vi "XNET Bus Monitor Redux.vi"() -> ()   [LabVIEW 2025, in "XNET Bus Monitor Client.lvlib"]
uses:
  XNET Bus Monitor Client.lvlib
  xnet_can_bus_monitor_api_client/RPC Messages/ni_xnet_can_bm_api_FrameFilter.ctl
  xnet_can_bus_monitor_api_client/RPC Messages/ni_xnet_can_bm_api_DirectionFilter.ctl
  Types/GUI.StateVariables.ctl
  Types/GUI.Controls.Refs.ctl
  Types/StreamEngine.QueueRefs.ctl
  Types/StreamEngine.CmdQueueData.ctl
  Types/StreamEngine.CmdQueueData.Cmd.ctl
  Types/SubProcessEngine.QueueRefs.ctl
  Types/SubProcessEngine.CmdQueueData.ctl
  Types/SubProcessEngine.CmdQueueData.Cmd.ctl
  Types/gRPC.ConnectionInfo.ctl
  <vilib>/gRPC/LabVIEW gRPC Library/Shared/grpcId.ctl
  Types/StreamEngine.State.ctl
  Types/SubProcessEngine.State.ctl
  Types/StreamEngine.CmdQueueData.InitialSettings.ctl
  xnet_can_bus_monitor_api_client/RPC Messages/ni_xnet_can_bm_api_StreamBusReply.ctl
  xnet_can_bus_monitor_api_client/RPC Messages/ni_xnet_can_bm_api_CanCommState.ctl
  xnet_can_bus_monitor_api_client/RPC Messages/ni_xnet_can_bm_api_CommState.ctl
  xnet_can_bus_monitor_api_client/RPC Messages/ni_xnet_can_bm_api_LastCommError.ctl
  xnet_can_bus_monitor_api_client/RPC Messages/ni_xnet_can_bm_api_Frame.ctl
  xnet_can_bus_monitor_api_client/RPC Messages/ni_xnet_can_bm_api_ErrorInfo.ctl
  Types/SubProcessEngine.CmdQueueData.Publish.ctl
  Types/StreamEngine.Parameters.ctl
  xnet_can_bus_monitor_api_client/RPC Messages/ni_xnet_can_bm_api_FilterInfo.ctl
  xnet_can_bus_monitor_api_client/RPC Messages/ni_xnet_can_bm_api_PassThruRequest.ctl
  xnet_can_bus_monitor_api_client/RPC Messages/ni_xnet_can_bm_api_SetStreamingFilterRequest.ctl
  <vilib>/Utility/miscctls.llb/LVRowAndColumnUnsignedTypeDef.ctl
  <vilib>/dlg_ctls.llb/Space Constant.vi
  SubVIs/Convert.BusDataArrayToStringArray.vi
  <vilib>/Utility/error.llb/Trim Whitespace.vi
  SubVIs/Convert.TimeToUTCString.vi
  <vilib>/Utility/error.llb/Trim Whitespace One-Sided.vi
  <vilib>/Utility/libraryn.llb/Check if File or Folder Exists.vi
  <vilib>/Utility/libraryn.llb/Get File Extension.vi
  <userlib>/_OpenG.lib/array/array.llb/Sort Array__ogtk.vi
  <userlib>/_OpenG.lib/array/array.llb/Sort 2D Array (String)__ogtk.vi
  xnet_can_bus_monitor_api_client/RPC Service/NI_XNET_CAN_Bus_Monitor_API/Begin NI_XNET_CAN_Bus_Monitor_API StreamBus.vi
  xnet_can_bus_monitor_api_client/RPC Service/NI_XNET_CAN_Bus_Monitor_API/End NI_XNET_CAN_Bus_Monitor_API StreamBus.vi
  xnet_can_bus_monitor_api_client/xnet_can_bus_monitor_api_client.lvlib
  <vilib>/gRPC/LabVIEW gRPC Library/grpc-lvsupport-release.lvlib
panel:
  out "error out":errorcluster
  out "Device":string
  in  "Tab Control":enum32{"Bus Stream", "RAW"}(tab)
  out "Log Status":string
  in  "Direction Filter":T1
  in  "Type Filter":T2
  in  "Reset Filter":bool
  in  "Host Filter":bool
  in  "Filter IDs":string caption="Filter IDs (format = x<ID>, comma separated, ID x0 = Bus Error)"
  in  "Clear History":bool
  out "Table Control":string[][](table)
  in  "Sort By ID":bool
  out "Stream Connected":bool
  out "Bus Status":string
  in  "Log":bool
  in  "Pause":bool
  in  "Extended?":bool
  in  "Identifier":u32 format="%x"
  in  "Raw Bytes":u8[](array[numeric])
  in  "Type":T3(ring)
  out "Error":errorcluster
  in  "Clear Raw":bool
  in  "Send Raw":bool
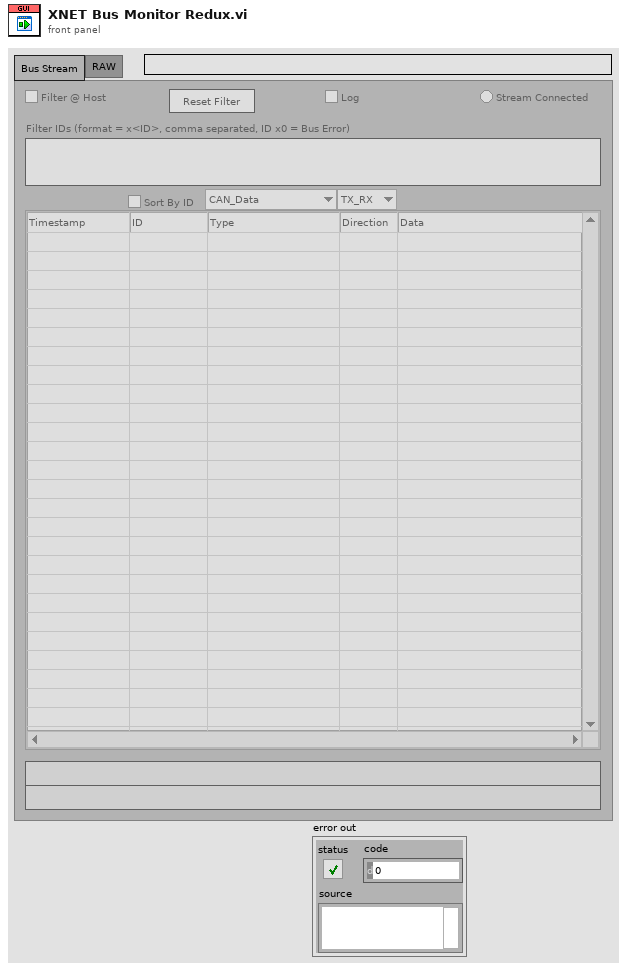
[diagram p1: front panel]
types:
  T1 = typedef "xnet_can_bus_monitor_api_client.lvlib/ni_xnet_can_bm_api_DirectionFilter.ctl" = enum32{"TX_RX", "RX", "TX"}
  T2 = typedef "xnet_can_bus_monitor_api_client.lvlib/ni_xnet_can_bm_api_FrameFilter.ctl" = enum32{"CAN_Data", "CAN_Remote", "CAN_Bus_Error", "CAN_2_Data", "CAN_FD_Data", "CAN_FD_BRS_Data", "J1939_Data", "Delay", "Log_Trigger", "Start_Trigger", "All"}
  T3 = enum16{"CAN Data", "CAN Remote", "CAN Bus Error", "CAN 2.0 Data", "CAN FD Data", "CAN FD+BRS Data", "J1939 Data", "Delay", "Log Trigger", "Start Trigger"}
  T4 = typedef "XNET Bus Monitor Client.lvlib/StreamEngine.CmdQueueData.InitialSettings.ctl" = cluster{"gRPC ID":T5, "Addon":string, "Project Folder":path}
  T5 = typedef "grpc-lvsupport-release.lvlib/grpcId.ctl" = u64
  T6 = typedef "XNET Bus Monitor Client.lvlib/SubProcessEngine.State.ctl" = enum8{"Idle", "Arm", "Process", "Stop", "Exit"}
  T7 = typedef "XNET Bus Monitor Client.lvlib/StreamEngine.State.ctl" = enum8{"Wait", "Start Stream", "Read Stream", "Stop Stream", "Exit"}
  T8 = typedef "XNET Bus Monitor Client.lvlib/GUI.StateVariables.ctl" = cluster{"UI.Refs":T9, "Connected?":bool, "Stream.Qs":T10, "Log Path":path, "gRPC Info":T12}
  T9 = typedef "XNET Bus Monitor Client.lvlib/GUI.Controls.Refs.ctl" = cluster{"Device":refnum<vi>, "Pause":refnum<vi>, "Table Control":refnum<vi>, "Sort By ID":refnum<vi>, "Streaming Connected":refnum<vi>, "Bus Status":refnum<vi>, "Direction Filter":refnum<vi>, "Type Filter":refnum<vi>, "Clear History":refnum<vi>, "Filter IDs":refnum<vi>, "Filter Location":refnum<vi>, "Reset Filter":refnum<vi>, "Log":refnum<vi>, "Type":refnum<vi>, "Extended?":refnum<vi>, "Identifier":refnum<vi>, "Raw Bytes":refnum<vi>, "Send Raw":refnum<vi>, "Clear Raw":refnum<vi>, "Raw Error":refnum<vi>, "Log Status":refnum<vi>}
  T10 = typedef "XNET Bus Monitor Client.lvlib/StreamEngine.QueueRefs.ctl" = cluster{"Cmd":refnum<queue>, "SubProcesses":T11}
  T11 = typedef "XNET Bus Monitor Client.lvlib/SubProcessEngine.QueueRefs.ctl" = cluster{"Process":refnum<queue>, "Log":refnum<queue>}
  T12 = typedef "XNET Bus Monitor Client.lvlib/gRPC.ConnectionInfo.ctl" = cluster{"IP Address":string, "Service Name":string, "Found Port":u64, "ID":T5}
  T13 = typedef "xnet_can_bus_monitor_api_client.lvlib/ni_xnet_can_bm_api_PassThruRequest.ctl" = cluster{"frame":T14}
  T14 = typedef "xnet_can_bus_monitor_api_client.lvlib/ni_xnet_can_bm_api_Frame.ctl" = cluster{"timestamp":dbl, "payload":u8[], "identifier":u32, "frame_type":u32, "extended":bool, "echo":bool}
  T15 = typedef "xnet_can_bus_monitor_api_client.lvlib/ni_xnet_can_bm_api_SetStreamingFilterRequest.ctl" = cluster{"filter_info":T16}
  T16 = typedef "xnet_can_bus_monitor_api_client.lvlib/ni_xnet_can_bm_api_FilterInfo.ctl" = cluster{"filter_ids":u32[], "direction_filter":T1, "frame_filter":T2}
  T17 = typedef "LVRowAndColumnUnsignedTypeDef.ctl" = cluster{"Row":u32, "Column":u32}
  T18 = typedef "xnet_can_bus_monitor_api_client.lvlib/ni_xnet_can_bm_api_StopProcessReply.ctl" = cluster{"stopped":bool, "error":T19}
  T19 = typedef "xnet_can_bus_monitor_api_client.lvlib/ni_xnet_can_bm_api_ErrorInfo.ctl" = errorcluster
  T20 = enum8{"Enabled", "Disabled", "Disabled and Grayed Out"}
  T21 = typedef "xnet_can_bus_monitor_api_client.lvlib/ni_xnet_can_bm_api_PassThruReply.ctl" = cluster{"error":T19}
  T22 = typedef "xnet_can_bus_monitor_api_client.lvlib/ni_xnet_can_bm_api_SetStreamingFilterReply.ctl" = cluster{"error":T19}
  T23 = typedef "xnet_can_bus_monitor_api_client.lvlib/ni_xnet_can_bm_api_ResetStreamingFilterReply.ctl" = cluster{"filter_info":T16, "error":T19}
  T24 = typedef "xnet_can_bus_monitor_api_client.lvlib/ni_xnet_can_bm_api_GetStreamingFilterReply.ctl" = cluster{"filter_info":T16, "error":T19}
  T25 = typedef "xnet_can_bus_monitor_api_client.lvlib/ni_xnet_can_bm_api_StreamBusReply.ctl" = cluster{"can_comm_state":T26, "frame":T14[], "error":T19}
  T26 = typedef "xnet_can_bus_monitor_api_client.lvlib/ni_xnet_can_bm_api_CanCommState.ctl" = cluster{"fault_code":i32, "fault":bool, "comm_state":T27, "last_comm_error":T28, "receive_error_counter":u32, "transmit_error_counter":u32, "transceiver_error":bool, "sleep":bool}
  T27 = typedef "xnet_can_bus_monitor_api_client.lvlib/ni_xnet_can_bm_api_CommState.ctl" = enum32{"Error_Active", "Error_Passive", "Bus_Off", "Init"}
  T28 = typedef "xnet_can_bus_monitor_api_client.lvlib/ni_xnet_can_bm_api_LastCommError.ctl" = enum32{"None", "Stuff", "Form", "ACK", "Bit1", "Bit0", "CRC"}
  T29 = typedef "XNET Bus Monitor Client.lvlib/SubProcessEngine.CmdQueueData.Publish.ctl" = cluster{"Response Data":T25, "Success":bool}
  T30 = typedef "XNET Bus Monitor Client.lvlib/SubProcessEngine.CmdQueueData.ctl" = cluster{"Cmd":T31, "Parameters":variant}
  T31 = typedef "XNET Bus Monitor Client.lvlib/SubProcessEngine.CmdQueueData.Cmd.ctl" = enum16{"Arm", "Publish", "Stop", "Exit"}
  T32 = typedef "XNET Bus Monitor Client.lvlib/StreamEngine.Parameters.ctl" = cluster{"Host Filter":bool, "Filter Parameters":T16, "Sort By ID":bool, "Pause":bool, "Clear History":bool}
  T33 = typedef "XNET Bus Monitor Client.lvlib/StreamEngine.CmdQueueData.ctl" = cluster{"Cmd":T34, "Parameters":variant}
  T34 = typedef "XNET Bus Monitor Client.lvlib/StreamEngine.CmdQueueData.Cmd.ctl" = enum8{"Start Stream", "Stop Stream", "Exit"}
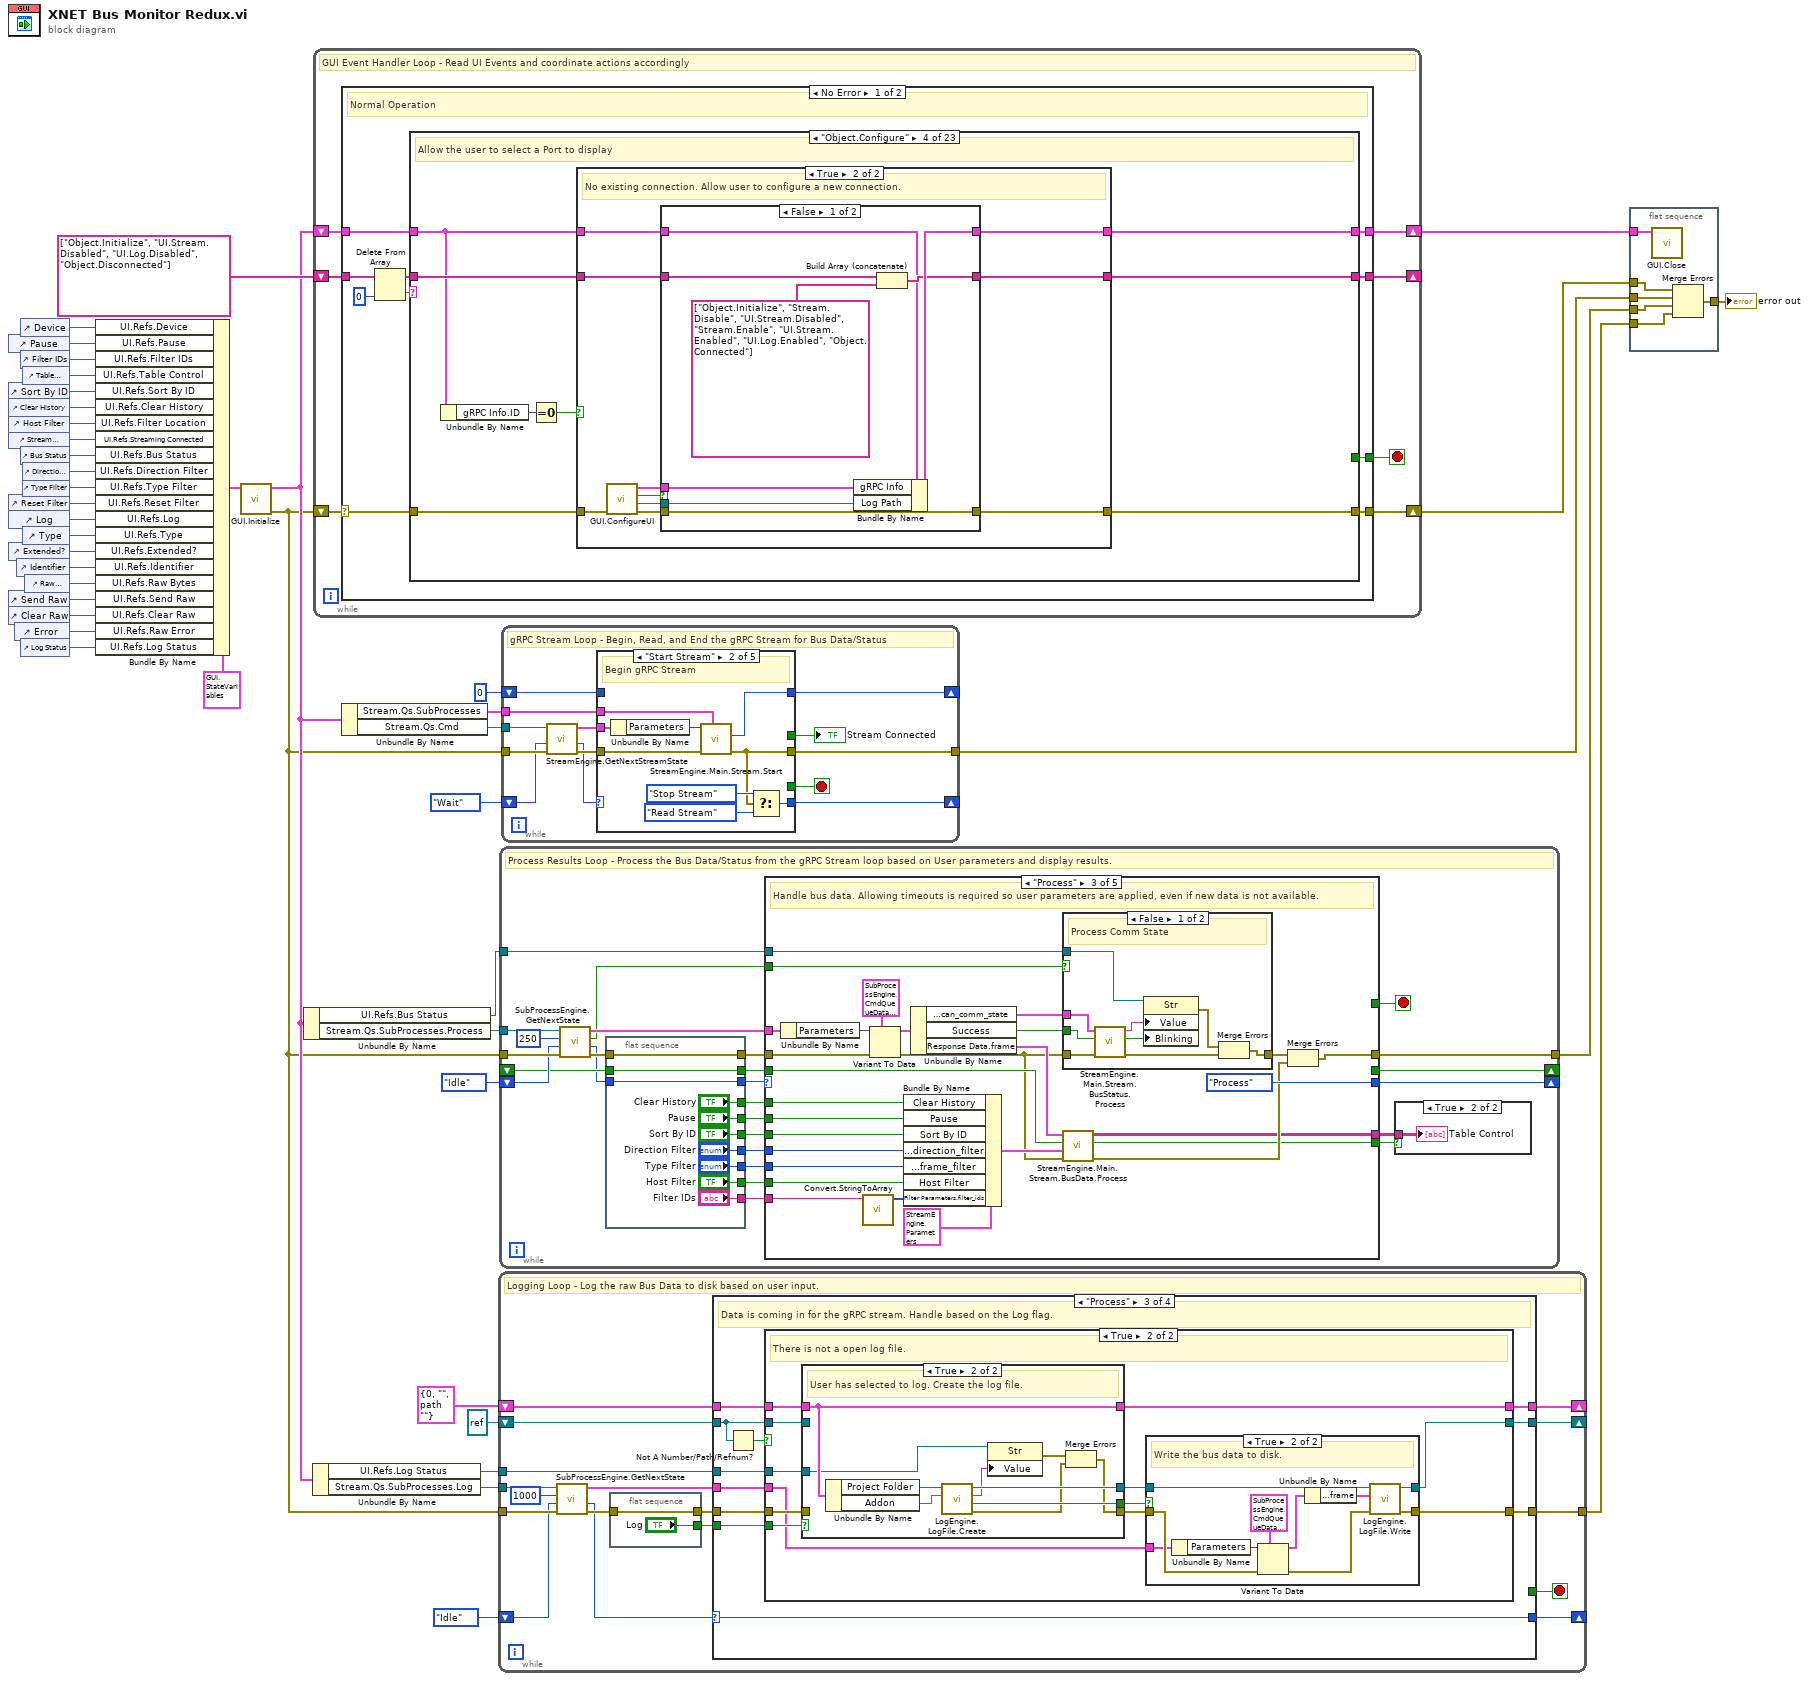
[diagram p0: block diagram]
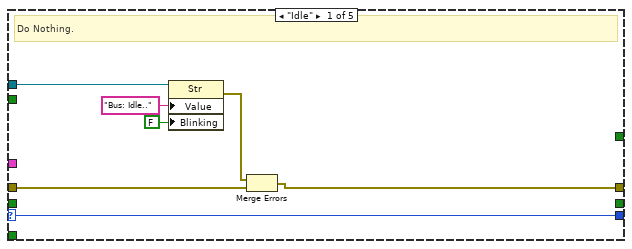
[diagram p3: hidden frame]
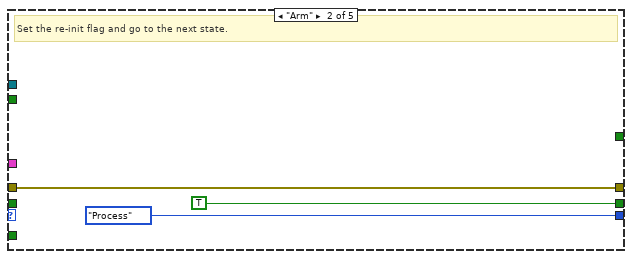
[diagram p4: hidden frame]
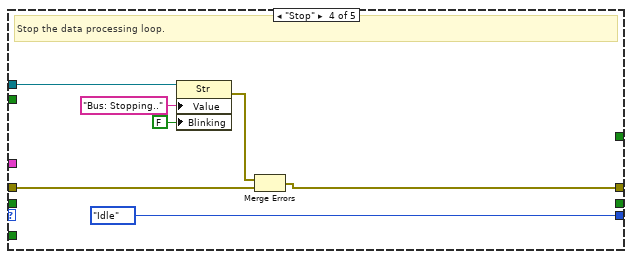
[diagram p6: hidden frame]
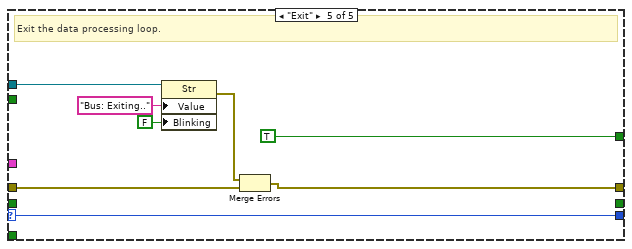
[diagram p7: hidden frame]
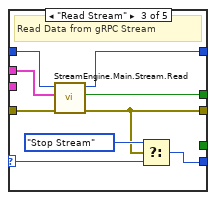
[diagram p9: hidden frame]
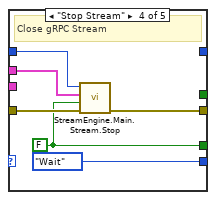
[diagram p10: hidden frame]
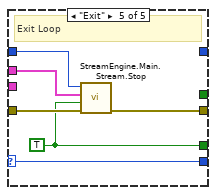
[diagram p11: hidden frame]
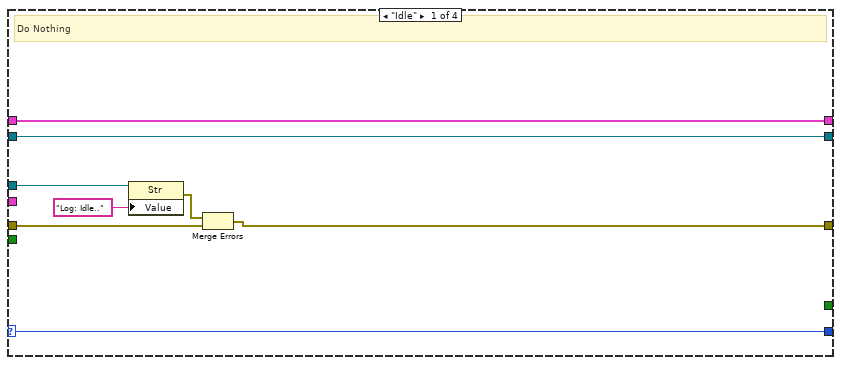
[diagram p12: hidden frame]
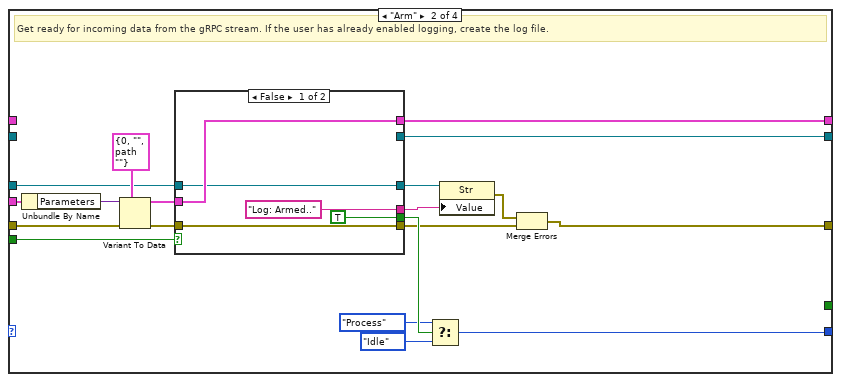
[diagram p13: hidden frame]
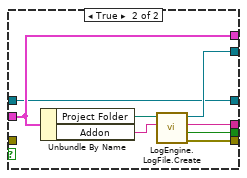
[diagram p14: hidden frame]
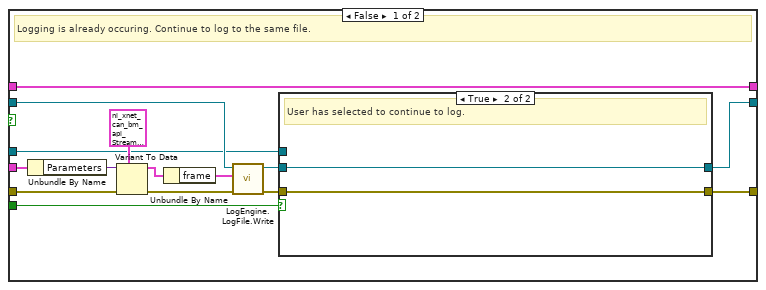
[diagram p15: hidden frame]
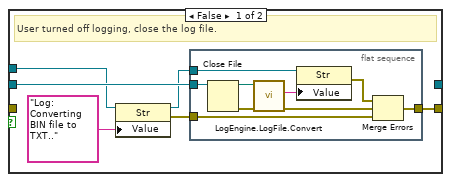
[diagram p16: hidden frame]
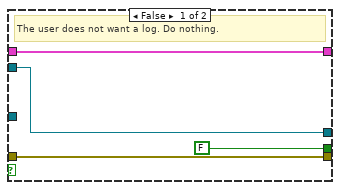
[diagram p18: hidden frame]
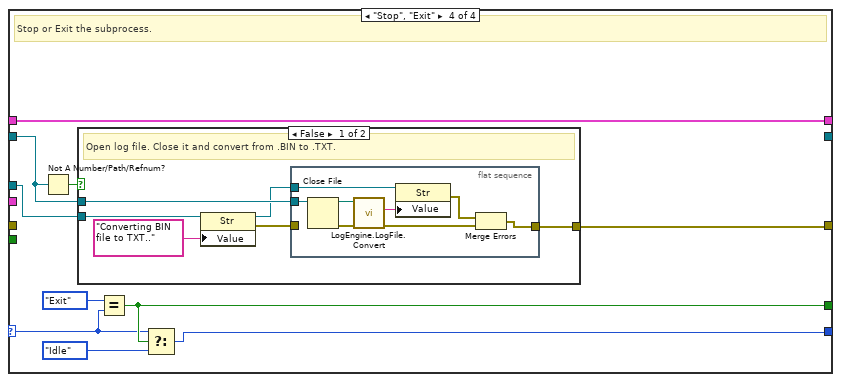
[diagram p19: hidden frame]
diagram:
  n1 = control-ref of="Pause"() -> (w21:refnum<vi>)
  n2 = control-ref of="Sort By ID"() -> (w40:refnum<vi>)
  n3 = control-ref of="Clear History"() -> (w36:refnum<vi>)
  n4 = control-ref of="Host Filter"() -> (w35:refnum<vi>)
  n5 = control-ref of="Stream Connected"() -> (w39:refnum<vi>)
  n6 = control-ref of="Reset Filter"() -> (w34:refnum<vi>)
  n7 = control-ref of="Log"() -> (w33:refnum<vi>)
  n8 = control-ref of="Extended?"() -> (w29:refnum<vi>)
  n9 = control-ref of="Send Raw"() -> (w26:refnum<vi>)
  n10 = control-ref of="Clear Raw"() -> (w27:refnum<vi>)
  n11 = control-ref of="Error"() -> (w28:refnum<vi>)
  n12 = control-ref of="Identifier"() -> (w30:refnum<vi>)
  n13 = control-ref of="Device"() -> (w23:refnum<vi>)
  n14 = control-ref of="Filter IDs"() -> (w37:refnum<vi>)
  n15 = control-ref of="Bus Status"() -> (w38:refnum<vi>)
  n16 = control-ref of="Log Status"() -> (w5:refnum<vi>)
  n17 = control-ref of="Table Control"() -> (w41:refnum<vi>)
  n18 = control-ref of="Direction Filter"() -> (w24:refnum<vi>)
  n19 = control-ref of="Type Filter"() -> (w25:refnum<vi>)
  n20 = control-ref of="Type"() -> (w32:refnum<vi>)
  n21 = control-ref of="Raw Bytes"() -> (w31:refnum<vi>)
  n22 = Bundle By Name(cluster=T8 {"UI.Refs"={"Device"=refnum, "Pause"=refnum, "Table Control"=refnum, "Sort By ID"=refnum, "Streaming Connected"=refnum, "Bus Status"=refnum, "Direction Filter"=refnum, "Type Filter"=refnum, "Clear History"=refnum, "Filter IDs"=refnum, "Filter Location"=refnum, "Reset Filter"=refnum, "Log"=refnum, "Type"=refnum, "Extended?"=refnum, "Identifier"=refnum, "Raw Bytes"=refnum, "Send Raw"=refnum, "Clear Raw"=refnum, "Raw Error"=refnum, "Log Status"=refnum}, "Connected?"=FALSE, "Stream.Qs"={"Cmd"=refnum, "SubProcesses"={"Process"=refnum, "Log"=refnum}}, "Log Path"=path "", "gRPC Info"={"IP Address"="", "Service Name"="", "Found Port"=0, "ID"=0}}, "UI.Refs.Device"=w23, "UI.Refs.Pause"=w21, "UI.Refs.Filter IDs"=w37, "UI.Refs.Table Control"=w41, "UI.Refs.Sort By ID"=w40, "UI.Refs.Clear History"=w36, "UI.Refs.Filter Location"=w35, "UI.Refs.Streaming Connected"=w39, "UI.Refs.Bus Status"=w38, "UI.Refs.Direction Filter"=w24, "UI.Refs.Type Filter"=w25, "UI.Refs.Reset Filter"=w34, "UI.Refs.Log"=w33, "UI.Refs.Type"=w32, "UI.Refs.Extended?"=w29, "UI.Refs.Identifier"=w30, "UI.Refs.Raw Bytes"=w31, "UI.Refs.Send Raw"=w26, "UI.Refs.Clear Raw"=w27, "UI.Refs.Raw Error"=w28, "UI.Refs.Log Status"=w5) -> (w22:T8)
  n23 = call "GUI.Initialize.vi"("State Variables in"=w22) -> ("error out"=w9:errorcluster, "State Variables out"=w12:T8)  [unwired: 9 in]
  n24 = Unbundle By Name(w12) -> ("UI.Refs.Bus Status"=w16:refnum<vi>, "Stream.Qs.SubProcesses.Process"=w17:refnum<queue>)
  n25 = Unbundle By Name(w12) -> ("UI.Refs.Log Status"=w4:refnum<vi>, "Stream.Qs.SubProcesses.Log"=w11:refnum<queue>)
  n26 = while {
    shift-right: [w49] -> _
    shift-left: string[] ["Object.Initialize", "UI.Stream.Disabled", "UI.Log.Disabled", "Object.Disconnected"] -> [w50]
    shift-right: [w47] -> w42
    shift-left: w12 -> [w46]
    shift-right: [w48] -> w7
    shift-left: w9 -> [w45]
    stop <- w51 stop-if-true
    # "GUI Event Handler Loop - Read UI Events and coordinate actions accordingly"
    n27 = case shown="No Error" w45 {
      selector: w45 -> [w52 w401]
      tunnel: [w61 _] -> w51
      tunnel: w50 -> [w59 w405]
      tunnel: [w56 w405] -> w49
      tunnel: [w55 w402] -> w48
      tunnel: [w54 w404] -> w47
      tunnel: w46 -> [w53 w404]
      frame No Error {
        # "Normal Operation"
        n28 = Delete From Array(array=w59, index=0) -> (deleted portion=w58:string, array with subset deleted=w57:string[])  [unwired: 1 in]
        n29 = case shown="\"Object.Configure\"" w58 {
          tunnel: [_ _ _ _ _ _ _ _ _ _ _ _ _ _ _ _ _ _ _ _ _ FALSE TRUE] -> w61
          tunnel: [w64 w70 w169 w177 w226 w234 w257 w259 w266 w280 w293 w306 w323 w327 w335 w348 w356 w368 w379 w385 w390 w396 w400] -> w56
          tunnel: w52 -> [w63 w68 w165 w175 w223 w231 w255 w261 w264 w277 w291 w303 w322 w326 w334 w346 w354 w366 w377 w380 w386 w393 w397]
          tunnel: w57 -> [w64 w69 w169 w176 w226 w234 w257 w258 w266 w280 w293 w306 w323 w327 w335 w348 w356 w368 w379 w385 w390 w396 w400]
          tunnel: w53 -> [w62 w65 w168 w173 w224 w228 w254 w262 w263 w279 w292 w305 w321 w325 w332 w347 w355 w367 w378 w384 w389 w392 w398]
          tunnel: [w63 w67 w161 w174 w213 w230 w245 w261 w265 w268 w290 w295 w322 w326 w333 w346 w354 w366 w377 w381 w387 w394 w397] -> w55
          tunnel: [w62 w66 w168 w178 w220 w229 w249 w262 w263 w279 w292 w305 w321 w325 w332 w347 w355 w367 w378 w384 w389 w392 w398] -> w54
          frame Default {
            # "Do nothing."
          }
          frame "" {
            # "Check for new events."
            n30 = event shown="[1] \"Send Raw\": Value Change" {
              selector: _ -> [_ _ _ _ _ _ _ _ _ _]
              dyn-events: _ -> [_ _ _ _ _ _ _ _ _ _]
              timeout: 250 -> [_ _ _ _ _ _ _ _ _ _]
              tunnel: [w72 w77 w86 w98 w109 w118 w128 w141 w150 w157] -> w70
              tunnel: w69 -> [w72 w78 w87 w97 w108 w117 w127 w140 w151 w158]
              tunnel: w68 -> [w74 w79 w88 w99 w110 w119 w129 w142 w154 w160]
              tunnel: [w74 w79 w88 w99 w110 w119 w129 w142 w154 w160] -> w67
              tunnel: [w73 w76 w85 w96 w107 w116 w126 w139 w153 w159] -> w66
              tunnel: w65 -> [w73 w76 w85 w96 w107 w116 w126 w139 w153 w159]
              event Timeout {
                # "No new events to be handled. Do Nothing."
                n31 = event-data() -> ()  [unwired: 2 out]
              }
              event "Send Raw": Value Change {
                # "User entered a new raw message and is ready to Send."
                n32 = event-data() -> ()  [unwired: 2 out]
                n33 = Unbundle By Name(w76) -> ("Connected?"=w75:bool)
                n34 = case shown="True" w75 {
                  tunnel: w78 -> [w80 w82]
                  tunnel: [w80 w81] -> w77
                  frame False {
                  }
                  frame True {
                    n35 = Build Array (concatenate)(w82, string[] ["Raw.Send"]) -> (w81:string[])
                  }
                }
              }
              event "Clear Raw": Value Change {
                # "The user has selected to clear all the values in the Raw tab."
                n36 = event-data() -> ()  [unwired: 2 out]
                n37 = Unbundle By Name(w85) -> ("Connected?"=w84:bool)
                n38 = case shown="True" w84 {
                  tunnel: w87 -> [w89 w91]
                  tunnel: [w89 w90] -> w86
                  frame False {
                  }
                  frame True {
                    n39 = Build Array (concatenate)(w91, string[] ["Raw.Clear"]) -> (w90:string[])
                  }
                }
              }
              event "Filter IDs": Value Change {
                # "The user has changed which IDs to filter. Apply changes."
                n40 = event-data() -> ()  [unwired: 2 out]
                n41 = Unbundle By Name(w96) -> ("Connected?"=w94:bool)
                n42 = local read "Host Filter"() -> (w95:bool)
                n43 = Compound Arithmetic op=AND(invert w95, w94) -> (w93:bool)
                n44 = case shown="False" w93 {
                  tunnel: w97 -> [w100 w104]
                  tunnel: [w101 w103] -> w98
                  frame False {
                    # "Handle filtering on the client/host."
                    n45 = Build Array (concatenate)(w100, "Stream.Table.GoUp") -> (w101:string[])
                  }
                  frame True {
                    # "Send updated filter parameters to Server."
                    n46 = Build Array (concatenate)(w104, string[] ["Stream.Filter.Send", "Stream.Table.GoUp"]) -> (w103:string[])
                  }
                }
              }
              event "Clear History", "Sort By ID": Value Change {
                # "The user has selected to make table changes. The processing loop will handle this but make the table go to the top."
                n47 = event-data() -> ()  [unwired: 2 out]
                n48 = Unbundle By Name(w107) -> ("Connected?"=w106:bool)
                n49 = case shown="True" w106 {
                  tunnel: [w111 w114] -> w109
                  tunnel: w108 -> [w111 w113]
                  frame False {
                  }
                  frame True {
                    n50 = Build Array (concatenate)(w113, "Stream.Table.GoUp") -> (w114:string[])
                  }
                }
              }
              event "Reset Filter": Value Change {
                # "The user has reset which IDs to filter. Apply changes."
                n51 = event-data() -> ()  [unwired: 2 out]
                n52 = Unbundle By Name(w116) -> ("Connected?"=w115:bool)
                n53 = case shown="True" w115 {
                  tunnel: w117 -> [w120 w122]
                  tunnel: [w120 w121] -> w118
                  frame False {
                  }
                  frame True {
                    n54 = Build Array (concatenate)(w122, string[] ["Stream.Filter.Reset", "Stream.Table.GoUp"]) -> (w121:string[])
                  }
                }
              }
              event "Host Filter": Value Change {
                # "The user has changed where filtering happens. Apply changes."
                n55 = event-data() -> ("NewVal"=w124:bool)  [unwired: 1 out]
                n56 = Unbundle By Name(w126) -> ("Connected?"=w125:bool)
                n57 = case shown="True" w125 {
                  tunnel: w127 -> [w130 w133]
                  tunnel: [w130 w132] -> w128
                  tunnel: w124 -> [_ w131]
                  frame False {
                  }
                  frame True {
                    n58 = case shown="True" w131 {
                      tunnel: [string[] ["Stream.Filter.Send", "Stream.Table.GoUp"] string[] ["Stream.Filter.Clear", "Stream.Table.GoUp"]] -> w134
                      frame False {
                      }
                      frame True {
                      }
                    }
                    n59 = Build Array (concatenate)(w133, w134) -> (w132:string[])
                  }
                }
              }
              event "Log": Value Change {
                # "Log loop will handle the logging but force the GUI to latch the configuration while a log session is occuring."
                n60 = event-data() -> ("NewVal"=w137:bool)  [unwired: 1 out]
                n61 = Unbundle By Name(w139) -> ("Connected?"=w138:bool)
                n62 = case shown="True" w138 {
                  tunnel: w140 -> [w143 w146]
                  tunnel: [w143 w145] -> w141
                  tunnel: w137 -> [_ w144]
                  frame False {
                  }
                  frame True {
                    n63 = case shown="False" w144 {
                      tunnel: [string[] ["UI.Log.Disabled"] string[] ["UI.Log.Enabled"]] -> w147
                      frame False {
                      }
                      frame True {
                      }
                    }
                    n64 = Build Array (concatenate)(w146, w147) -> (w145:string[])
                  }
                }
              }
              event Menu Selection (User) {
                # "Queue up the Configure or Exit commands from the run time menu."
                n65 = event-data() -> ("ItemTag"=w152:string)  [unwired: 1 out]
                n66 = Build Array (concatenate)(w151, w152) -> (w150:string[])
              }
              event Panel Close? {
                # "Discard the user panel close and handle nicely."
                n67 = event-data() -> ()  [unwired: 5 out]
                n68 = Build Array (concatenate)(w158, "Object.Exit") -> (w157:string[])
                n69 = event-data("Discard?"=TRUE) -> ()  [unwired: 1 in, 1 out]
              }
            }
          }
          frame "Object.Initialize" {
            # "Initialize the GUI"
            n70 = Unbundle By Name(w168) -> ("UI.Refs.Device"=w163:refnum<vi>, "UI.Refs.Filter Location"=w166:refnum<vi>)
            n71 = property class="Bool (strict)"(reference=w166, error in=w165, "Value"=FALSE) -> (error out=w162:errorcluster)  [unwired: 1 out]
            n72 = local write "Tab Control"(0) -> ()
            n73 = property class="Str"(reference=w163, error in=w162, "Value"="Initializing!!") -> (error out=w161:errorcluster)  [unwired: 1 out]
          }
          frame "Object.Configure" {
            # "Allow the user to select a Port to display"
            n74 = Unbundle By Name(w173) -> ("gRPC Info.ID"=w172:T5)
            n75 = Equal To 0?(x=w172) -> (x = 0?=w171:bool)
            n76 = case shown="True" w171 {
              tunnel: [w180 w200] -> w178
              tunnel: [w179 w199] -> w177
              tunnel: w176 -> [w182 w198]
              tunnel: w175 -> [w186 w195]
              tunnel: [w186 w194] -> w174
              tunnel: w173 -> [w181 w191]
              frame False {
                # "A connection already exists. Ask the user if they want to close it."
                n77 = Two Button Dialog(message="Configuring will close the current session. Continue?", 2:"Yes" ("T button name (\"OK\")")) -> (T button?=w183:bool)  [unwired: 1 in]
                n78 = case shown="True" w183 {
                  tunnel: w182 -> [w187 _]
                  tunnel: w181 -> [w188 w190]
                  tunnel: [w188 w190] -> w180
                  tunnel: [w187 string[] ["Stream.Disable", "UI.Stream.Disabled", "UI.Log.Disabled", "Object.Disconnect", "Object.Disconnected", "Object.Initialize", "Object.Configure"]] -> w179
                  frame False {
                  }
                  frame True {
                  }
                }
              }
              frame True {
                # "No existing connection. Allow user to configure a new connection."
                n79 = call "GUI.ConfigureUI.vi"("error in (no error)"=w195) -> ("error out"=w193:errorcluster, "Log Path out"=w192:path, "Canceled?"=w197:bool, "gRPC Info"=w196:T12)  [unwired: 7 in]
                n80 = case shown="False" w197 {
                  tunnel: w191 -> [w203 w210]
                  tunnel: [w208 w210] -> w200
                  tunnel: [w206 w211] -> w199
                  tunnel: w198 -> [w207 w211]
                  tunnel: w196 -> [w204 _]
                  tunnel: [w202 w209] -> w194
                  tunnel: w193 -> [w202 w209]
                  tunnel: w192 -> [w201 _]
                  frame False {
                    n81 = Bundle By Name(cluster=w203, "gRPC Info"=w204, "Log Path"=w201) -> (w208:T8)
                    n82 = Build Array (concatenate)(w207, string[] ["Object.Initialize", "Stream.Disable", "UI.Stream.Disabled", "Stream.Enable", "UI.Stream.Enabled", "UI.Log.Enabled", "Object.Connected"]) -> (w206:string[])
                  }
                  frame True {
                    # "User canceled"
                  }
                }
              }
            }
          }
          frame "Object.Connected" {
            # "gRPC connected. Update the GUI accordingly."
            n83 = call "GUI.DisableState.Set.vi"("Enable?"=TRUE, "error in (no error)"=w223, "State Variables in"=w224) -> ("error out"=w219:errorcluster, "State Variables out"=w221:T8)  [unwired: 7 in]
            n84 = Unbundle By Name(w221) -> ("UI.Refs.Log"=w215:refnum<vi>, "Log Path"=w216:path, "UI.Refs.Device"=w218:refnum<vi>, "gRPC Info.Service Name"=w217:string)
            n85 = property class="Str"(reference=w218, error in=w219, "Value"=w217) -> (error out=w214:errorcluster)  [unwired: 1 out]
            n86 = call <vilib>:"Is Path and Not Empty.vi"("path"=w216) -> ("Is Path and Not Empty?"=w212:bool)  [unwired: 4 in]
            n87 = property class="Bool (strict)"(reference=w215, error in=w214, "Visible"=w212) -> (error out=w213:errorcluster)  [unwired: 1 out]
            n88 = Bundle By Name(cluster=w221, "Connected?"=TRUE) -> (w220:T8)
          }
          frame "Object.Disconnect" {
            # "Disconnect from the Server."
            n89 = Unbundle By Name(w228) -> ("gRPC Info.ID"=w232:T5)
            n90 = Equal To 0?(x=w232) -> (x = 0?=w233:bool)
            n91 = case shown="False" w233 {
              tunnel: w232 -> [w241 _]
              tunnel: w231 -> [w238 w243]
              tunnel: [w238 w243] -> w230
              frame False {
                n92 = call "NI_XNET_CAN_Bus_Monitor_API StopProcess.vi"("gRPC ID"=w241) -> ("error out"=w236:errorcluster, "Response Data"=w237:T18, "gRPC ID out"=w242:T5)  [unwired: 8 in]
                n93 = call "gRPC.Response.GetError.vi"("error in (no error)"=w236, "Response"=w237) -> ("error out"=w235:errorcluster)  [unwired: 9 in]
                n94 = call "Destroy Client.vi"("gRPC ID"=w242) -> ("error out"=w240:errorcluster)  [unwired: 10 in]
                n95 = Merge Errors(w235, w240) -> (w239:errorcluster)
                n96 = call <vilib>:"Simple Error Handler.vi"("error in (no error)"=w239) -> ()  [unwired: 4 in, 5 out]
              }
              frame True {
              }
            }
            n97 = Bundle By Name(cluster=w228, "gRPC Info"=T12 {"IP Address"="", "Service Name"="", "Found Port"=0, "ID"=0}) -> (w229:T8)
          }
          frame "Object.Disconnected" {
            # "Disconnected from the Server. Update the GUI accordingly."
            n98 = call "GUI.DisableState.Set.vi"("Enable?"=FALSE, "error in (no error)"=w255, "State Variables in"=w254) -> ("error out"=w251:errorcluster, "State Variables out"=w250:T8)  [unwired: 7 in]
            n99 = Unbundle By Name(w250) -> ("UI.Refs.Log"=w247:refnum<vi>, "UI.Refs.Device"=w252:refnum<vi>)
            n100 = property class="Str"(reference=w252, error in=w251, "Value"="Object Disconnected - Configure") -> (error out=w246:errorcluster)  [unwired: 1 out]
            n101 = property class="Bool (strict)"(reference=w247, error in=w246, "Visible"=TRUE ("Value")) -> (error out=w245:errorcluster)  [unwired: 1 out]
            n102 = Bundle By Name(cluster=w250, "Connected?"=FALSE) -> (w249:T8)
          }
          frame "Object.Exit" {
            # "Queue all the commands to cleanly exit."
            n103 = Build Array (concatenate)(w258, string[] ["Stream.Disable", "UI.Stream.Disabled", "UI.Log.Disabled", "Object.Disconnect", "Object.Disconnected", "Stream.Exit", "App.Exit"]) -> (w259:string[])
          }
          frame "UI.Stream.Enabled" {
            n104 = call "GUI.Stream.Enable.vi"("error in (no error)"=w264, "State Variables in"=w263) -> ("error out"=w265:errorcluster)  [unwired: 9 in]
          }
          frame "UI.Log.Enabled" {
            w267 = T20."Disabled and Grayed Out" ("Disabled")
            # "Logging has be enabled. Stop the user from changing filter settings so that the data coming from the Server is the same."
            n105 = Unbundle By Name(w279) -> ("UI.Refs.Type Filter"=w272:refnum<vi>, "UI.Refs.Filter IDs"=w271:refnum<vi>, "UI.Refs.Direction Filter"=w270:refnum<vi>, "UI.Refs.Reset Filter"=w275:refnum<vi>, "UI.Refs.Filter Location"=w278:refnum<vi>)
            n106 = property class="Bool (strict)"(reference=w278, error in=w277, "DisabledEnum"=w267) -> (error out=w276:errorcluster, "Value"=w274:bool)  [unwired: 1 out]
            n107 = Build Array(w272, w271, w270) -> (w269:refnum<vi>[])
            n108 = property class="Bool"(reference=w275, error in=w276, "DisabledEnum"=w267) -> (error out=w273:errorcluster)  [unwired: 1 out]
            n109 = case shown="False" w274 {
              tunnel: w273 -> [w283 w289]
              tunnel: w269 -> [w284 _]
              tunnel: [w282 w289] -> w268
              tunnel: w267 -> [w281 _]
              frame False {
                n110 = for {
                  tunnel: w284 -> [w288] mode=indexing
                  shift-right: [w286] -> w282
                  shift-left: w283 -> [w287]
                  tunnel: w281 -> [w285]
                  n111 = property class="Ctl"(reference=w288, error in=w287, "DisabledEnum"=w285) -> (error out=w286:errorcluster)  [unwired: 1 out]
                }
              }
              frame True {
              }
            }
          }
          frame "UI.Stream.Disabled" {
            n112 = call "GUI.Stream.Disable.vi"("error in (no error)"=w291, "State Variables in"=w292) -> ("error out"=w290:errorcluster)  [unwired: 9 in]
          }
          frame "UI.Log.Disabled" {
            w294 = T20."Enabled" ("Disabled")
            # "Logging has been turned off so re-enable the filter options."
            n113 = Unbundle By Name(w305) -> ("UI.Refs.Type Filter"=w299:refnum<vi>, "UI.Refs.Filter IDs"=w298:refnum<vi>, "UI.Refs.Direction Filter"=w297:refnum<vi>, "UI.Refs.Reset Filter"=w301:refnum<vi>, "UI.Refs.Filter Location"=w304:refnum<vi>)
            n114 = property class="Bool (strict)"(reference=w304, error in=w303, "DisabledEnum"=w294) -> (error out=w302:errorcluster)  [unwired: 1 out]
            n115 = Build Array(w299, w298, w297) -> (w296:refnum<vi>[])
            n116 = property class="Bool"(reference=w301, error in=w302, "DisabledEnum"=w294) -> (error out=w300:errorcluster)  [unwired: 1 out]
            n117 = for {
              tunnel: w296 -> [w310] mode=indexing
              shift-right: [w308] -> w295
              shift-left: w300 -> [w309]
              tunnel: w294 -> [w307]
              n118 = property class="Ctl"(reference=w310, error in=w309, "DisabledEnum"=w307) -> (error out=w308:errorcluster)  [unwired: 1 out]
            }
          }
          frame "Raw.Send" {
            # "Send a raw frame to be put directly on the bus."
            n119 = Bundle By Name(cluster=T13 {"frame"={"timestamp"=0.0, "payload"=[], "identifier"=0, "frame_type"=0, "extended"=FALSE, "echo"=FALSE}} ("Request Data"), "frame.extended"="Extended?", "frame.frame_type"="Type", "frame.identifier"="Identifier", "frame.payload"="Raw Bytes") -> (w315:T13)
            n120 = Unbundle By Name(w321) -> ("gRPC Info.ID"=w314:T5)
            n121 = call "NI_XNET_CAN_Bus_Monitor_API PassThru.vi"("Request Data"=w315, "gRPC ID"=w314) -> ("error out"=w312:errorcluster, "Response Data"=w313:T21)  [unwired: 7 in, 1 out]
            n122 = call "gRPC.Response.GetError.vi"("error in (no error)"=w312, "Response"=w313) -> ("error out"=→"Error":errorcluster)  [unwired: 9 in]
          }
          frame "Raw.Clear" {
            # "Clear the raw bytes GUI."
            n123 = local write "Raw Bytes"(u8[] [] ("Cmd")) -> ()
          }
          frame "Stream.Enable" {
            # "Start the gRPC stream loop."
            n124 = Unbundle By Name(w332) -> ("Stream.Qs"=w331:T10, "gRPC Info.ID"=w330:T5, "gRPC Info.Service Name"=w329:string, "Log Path"=w328:path)
            n125 = call "StreamEngine.StartCmd.Send.vi"("Project Folder"=w328, "error in (no error)"=w334, "Addon"=w329, "gRPC ID"=w330, "Q Refs"=w331) -> ("error out"=w333:errorcluster)  [unwired: 6 in]
          }
          frame "Stream.Filter.Send" {
            # "Send a filter update to the server."
            n126 = local read "Direction Filter"() -> (w344:T1)
            n127 = local read "Type Filter"() -> (w343:T2)
            n128 = local read "Filter IDs"() -> (w345:string)
            n129 = Unbundle By Name(w347) -> ("gRPC Info.ID"=w339:T5)
            n130 = call "Convert.StringToArray.vi"("Filter IDs"=w345) -> ("Filter IDs"=w342:u32[])  [unwired: 10 in]
            n131 = Bundle By Name(cluster=T15 {"filter_info"={"filter_ids"=[], "direction_filter"=enum."TX_RX", "frame_filter"=enum."CAN_Data"}} ("Request Data"), "filter_info.frame_filter"=w343, "filter_info.direction_filter"=w344, "filter_info.filter_ids"=w342) -> (w340:T15)
            n132 = call "NI_XNET_CAN_Bus_Monitor_API SetStreamingFilter.vi"("Request Data"=w340, "gRPC ID"=w339) -> ("error out"=w338:errorcluster, "Response Data"=w336:T22)  [unwired: 7 in, 1 out]
            n133 = call "gRPC.Response.GetError.vi"("error in (no error)"=w338, "Response"=w336) -> ("error out"=w337:errorcluster)  [unwired: 9 in]
            n134 = call <vilib>:"Simple Error Handler.vi"("error in (no error)"=w337) -> ()  [unwired: 4 in, 5 out]
          }
          frame "Stream.Filter.Clear" {
            # "Command the server to clear out the filters."
            n135 = Unbundle By Name(w355) -> ("gRPC Info.ID"=w352:T5)
            n136 = call "NI_XNET_CAN_Bus_Monitor_API SetStreamingFilter.vi"("Request Data"=T15 {"filter_info"={"filter_ids"=[], "direction_filter"=enum."TX_RX", "frame_filter"=enum."CAN_Data"}}, "gRPC ID"=w352) -> ("error out"=w350:errorcluster, "Response Data"=w351:T22)  [unwired: 7 in, 1 out]
            n137 = call "gRPC.Response.GetError.vi"("error in (no error)"=w350, "Response"=w351) -> ("error out"=w349:errorcluster)  [unwired: 9 in]
            n138 = call <vilib>:"Simple Error Handler.vi"("error in (no error)"=w349) -> ()  [unwired: 4 in, 5 out]
          }
          frame "Stream.Filter.Reset" {
            # "Send a command to the server to reset the filter back to the default configuration."
            n139 = Unbundle By Name(w367) -> ("gRPC Info.ID"=w360:T5)
            n140 = call "NI_XNET_CAN_Bus_Monitor_API ResetStreamingFilter.vi"("gRPC ID"=w360) -> ("error out"=w358:errorcluster, "Response Data"=w359:T23)  [unwired: 8 in, 1 out]
            n141 = Unbundle By Name(w359) -> ("filter_info.filter_ids"=w362:u32[], "filter_info.direction_filter"=w364:T1, "filter_info.frame_filter"=w363:T2)
            n142 = call "gRPC.Response.GetError.vi"("error in (no error)"=w358, "Response"=w359) -> ("error out"=w357:errorcluster)  [unwired: 9 in]
            n143 = call <vilib>:"Simple Error Handler.vi"("error in (no error)"=w357) -> ()  [unwired: 4 in, 5 out]
            n144 = local write "Host Filter"(FALSE ("Host Filter")) -> ()
            n145 = call "Convert.ArrayToString.vi"("Filter IDs"=w362) -> ("Filter IDs"=w361:string)  [unwired: 10 in]
            n146 = local write "Filter IDs"(w361) -> ()
            n147 = local write "Direction Filter"(w364) -> ()
            n148 = local write "Type Filter"(w363) -> ()
          }
          frame "Stream.Filter.Read" {
            # "Get the current filter settings from the Server."
            n149 = Unbundle By Name(w378) -> ("gRPC Info.ID"=w372:T5)
            n150 = call "NI_XNET_CAN_Bus_Monitor_API GetStreamingFilter.vi"("gRPC ID"=w372) -> ("error out"=w371:errorcluster, "Response Data"=w370:T24)  [unwired: 8 in, 1 out]
            n151 = Unbundle By Name(w370) -> ("filter_info.filter_ids"=w374:u32[], "filter_info.direction_filter"=w376:T1, "filter_info.frame_filter"=w375:T2)
            n152 = call "gRPC.Response.GetError.vi"("error in (no error)"=w371, "Response"=w370) -> ("error out"=w369:errorcluster)  [unwired: 9 in]
            n153 = call <vilib>:"Simple Error Handler.vi"("error in (no error)"=w369) -> ()  [unwired: 4 in, 5 out]
            n154 = call "Convert.ArrayToString.vi"("Filter IDs"=w374) -> ("Filter IDs"=w373:string)  [unwired: 10 in]
            n155 = local write "Filter IDs"(w373) -> ()
            n156 = local write "Direction Filter"(w376) -> ()
            n157 = local write "Type Filter"(w375) -> ()
          }
          frame "Stream.Table.GoUp" {
            # "Go to the top of the bus table. This is needed for when filters are applied and the user has scrolled down in the list."
            n158 = Unbundle By Name(w384) -> ("UI.Refs.Table Control"=w382:refnum<vi>)
            n159 = property class="Tbl (strict)"(reference=w382, error in=w380, "Index Values"=T17 {"Row"=0, "Column"=0}) -> (error out=w381:errorcluster)  [unwired: 1 out]
          }
          frame "Stream.Disable" {
            # "Stop the gRPC stream to the Server."
            n160 = Unbundle By Name(w389) -> ("Stream.Qs"=w388:T10)
            n161 = call "StreamEngine.StopCmd.Send.vi"("error in (no error)"=w386, "Q Refs"=w388) -> ("error out"=w387:errorcluster)  [unwired: 9 in]
          }
          frame "Stream.Exit" {
            # "Tell the gRPC stream loop to exit."
            n162 = Unbundle By Name(w392) -> ("Stream.Qs"=w391:T10)
            n163 = call "StreamEngine.ExitCmd.Send.vi"("error in (no error)"=w393, "Q Refs"=w391) -> ("error out"=w394:errorcluster)  [unwired: 9 in]
          }
          frame "App.Exit" {
            # "Stop the GUI Event Handler (this) Loop."
          }
        }
      }
      frame Error {
        # "Handle Errors."
        n164 = call <vilib>:"Simple Error Handler.vi"("error in (no error)"=w401) -> ("error out"=w403:errorcluster)  [unwired: 4 in, 4 out]
        n165 = call <vilib>:"Clear Errors.vi"("error in (no error)"=w403) -> ("error out"=w402:errorcluster)  [unwired: 5 in, 1 out]
      }
    }
  }
  n166 = Unbundle By Name(w12) -> ("Stream.Qs.SubProcesses"=w14:T11, "Stream.Qs.Cmd"=w19:refnum<queue>)
  n167 = while {
    tunnel: w11 -> [w422]
    shift-right: [w417] -> _
    shift-left: SubProcessEngine.State."Idle" ("State") -> [w408]
    tunnel: w9 -> [w421]
    shift-right: [w420] -> _
    shift-left: refnum<file> refnum ("Byte Stream File out") -> [w419]
    shift-right: [w415] -> _
    shift-left: T4 {"gRPC ID"=0, "Addon"="", "Project Folder"=path ""} ("cluster") -> [w414]
    tunnel: [w410] -> w6
    tunnel: w4 -> [w409]
    stop <- w416 stop-if-true
    # "Logging Loop - Log the raw Bus Data to disk based on user input."
    n168 = call "SubProcessEngine.GetNextState.vi"("error in (no error)"=w421, "State"=w408, "timeout in ms (5)"=1000, "Q"=w422) -> ("error out"=w412:errorcluster, "State"=w406:T6, "Data"=w418:T30)  [unwired: 4 in, 1 out]
    n169 = flat-sequence {
      tunnel: ["Log"] -> w413
      tunnel: w412 -> [w423]
      tunnel: [w423] -> w411
      frame #0 {
      }
    }
    n170 = case shown="\"Process\"" w406 {
      selector: w406 -> [w431 _ w466 w547]
      tunnel: [w432 w444 w474 _] -> w420
      tunnel: w419 -> [w432 _ w473 w554]
      tunnel: [w426 w436 w475 w546] -> w410
      tunnel: w411 -> [w427 w448 w468 _]
      tunnel: w418 -> [_ w451 w467 _]
      tunnel: [w431 w440 w466 w548] -> w417
      tunnel: [_ _ _ w551] -> w416
      tunnel: [w430 w446 w471 w553] -> w415
      tunnel: w414 -> [w430 _ w472 w553]
      tunnel: w413 -> [_ w439 w470 _]
      tunnel: w409 -> [w429 w434 w465 w552]
      frame "Idle" {
        # "Do Nothing"
        n171 = property class="Str"(reference=w429, "Value"="Log: Idle..") -> (error out=w428:errorcluster)  [unwired: 1 in, 1 out]
        n172 = Merge Errors(w428, w427) -> (w426:errorcluster)
      }
      frame "Arm" {
        # "Get ready for incoming data from the gRPC stream. If the user has already enabled logging, create the log file."
        n173 = Unbundle By Name(w451) -> ("Parameters"=w450:variant)
        n174 = Variant To Data(error in=w448, type=T4 {"gRPC ID"=0, "Addon"="", "Project Folder"=path ""} ("cluster"), Variant=w450) -> (data=w447:T4, error out=w445:errorcluster)
        n175 = case shown="False" w439 {
          tunnel: ["Log: Armed.." ("Status") w462] -> w437
          tunnel: [w456 w461] -> w435
          tunnel: w445 -> [w456 _]
          tunnel: [TRUE ("Continue") w460] -> w443
          tunnel: w447 -> [w454 w459]
          tunnel: [w454 w459] -> w446
          tunnel: [_ w458] -> w444
          tunnel: w434 -> [w452 w457]
          tunnel: [w452 w457] -> w433
          frame False {
          }
          frame True {
            n176 = Unbundle By Name(w459) -> ("Project Folder"=w464:path, "Addon"=w463:string)
            n177 = call "LogEngine.LogFile.Create.vi"("Port"=w463, "Project Folder"=w464) -> ("error out"=w461:errorcluster, "Continue"=w460:bool, "Status"=w462:string, "Byte Stream File out"=w458:refnum<file>)  [unwired: 6 in]
          }
        }
        n178 = Select(t=SubProcessEngine.State."Process" ("State"), s=w443, f=SubProcessEngine.State."Idle") -> (s? t:f=w440:T6)
        n179 = property class="Str"(reference=w433, "Value"=w437) -> (error out=w438:errorcluster)  [unwired: 1 in, 1 out]
        n180 = Merge Errors(w438, w435) -> (w436:errorcluster)
      }
      frame "Process" {
        # "Data is coming in for the gRPC stream. Handle based on the Log flag."
        n181 = Not A Number/Path/Refnum?(number/path/refnum=w473) -> (NaN/Path/Refnum?=w469:bool)
        n182 = case shown="True" w469 {
          tunnel: [w476 w508] -> w475
          tunnel: [w477 w517] -> w474
          tunnel: w473 -> [w488 w516]
          tunnel: w472 -> [w490 w514]
          tunnel: [w490 w513] -> w471
          tunnel: w470 -> [w480 w512]
          tunnel: w468 -> [w489 w511]
          tunnel: w467 -> [w482 w510]
          tunnel: w465 -> [w478 w509]
          frame False {
            # "Logging is already occuring. Continue to log to the same file."
            n183 = Unbundle By Name(w482) -> ("Parameters"=w485:variant)
            n184 = Variant To Data(error in=w489, type=T25 {"can_comm_state"={"fault_code"=0, "fault"=FALSE, "comm_state"=enum."Error_Active", "last_comm_error"=enum."None", "receive_error_counter"=0, "transmit_error_counter"=0, "transceiver_error"=FALSE, "sleep"=FALSE}, "frame"=[], "error"={"status"=FALSE, "code"=0, "source"=""}} ("Response Data"), Variant=w485) -> (data=w484:T25, error out=w487:errorcluster)
            n185 = Unbundle By Name(w484) -> ("frame"=w483:T14[])
            n186 = call "LogEngine.LogFile.Write.vi"("error in (no error)"=w487, "Data"=w483, "Byte Stream File in"=w488) -> ("error out"=w479:errorcluster, "Byte Stream File out"=w481:refnum<file>)  [unwired: 7 in]
            n187 = case shown="True" w480 {
              tunnel: w481 -> [w496 w506]
              tunnel: [w492 w507] -> w476
              tunnel: w478 -> [w495 _]
              tunnel: w479 -> [_ w507]
              tunnel: [_ w506] -> w477
              frame False {
                # "User turned off logging, close the log file."
                n188 = property class="Str"(reference=w495, "Value"="Log: Converting BIN file to TXT..") -> (reference out=w493:refnum<vi>, error out=w491:errorcluster)  [unwired: 1 in]
                n189 = flat-sequence {
                  tunnel: w496 -> [w505]
                  tunnel: w493 -> [w501]
                  tunnel: [w499] -> w492
                  tunnel: w491 -> [w497]
                  frame #0 {
                    n190 = Close File(refnum=w505) -> (path=w504:path, error out=w503:errorcluster)  [unwired: 1 in]
                    n191 = call "LogEngine.LogFile.Convert.vi"("error in (no error)"=w503, "path"=w504) -> ("error out"=w498:errorcluster, "Status"=w500:string)  [unwired: 8 in]
                    n192 = property class="Str"(reference=w501, "Value"=w500) -> (error out=w502:errorcluster)  [unwired: 1 in, 1 out]
                    n193 = Merge Errors(w502, w498, w497) -> (w499:errorcluster)
                  }
                }
              }
              frame True {
                # "User has selected to continue to log."
              }
            }
          }
          frame True {
            # "There is not a open log file."
            n194 = case shown="True" w512 {
              tunnel: [w534 w536] -> w519
              tunnel: [w535 w543] -> w518
              tunnel: w516 -> [w535 _]
              tunnel: [FALSE ("Continue") w542] -> w515
              tunnel: w511 -> [w534 _]
              tunnel: w514 -> [w533 w541]
              tunnel: [w533 w541] -> w513
              tunnel: w509 -> [_ w539]
              frame False {
                # "The user does not want a log. Do nothing."
              }
              frame True {
                # "User has selected to log. Create the log file."
                n195 = Unbundle By Name(w541) -> ("Project Folder"=w545:path, "Addon"=w544:string)
                n196 = call "LogEngine.LogFile.Create.vi"("Port"=w544, "Project Folder"=w545) -> ("error out"=w537:errorcluster, "Continue"=w542:bool, "Status"=w538:string, "Byte Stream File out"=w543:refnum<file>)  [unwired: 6 in]
                n197 = property class="Str"(reference=w539, "Value"=w538) -> (error out=w540:errorcluster)  [unwired: 1 in, 1 out]
                n198 = Merge Errors(w540, w537) -> (w536:errorcluster)
              }
            }
            n199 = case shown="True" w515 {
              tunnel: w519 -> [w520 w527]
              tunnel: w518 -> [w521 w531]
              tunnel: [w520 w530] -> w508
              tunnel: [w521 w529] -> w517
              tunnel: w510 -> [_ w526]
              frame False {
                # "Do nothing."
              }
              frame True {
                # "Write the bus data to disk."
                n200 = Unbundle By Name(w526) -> ("Parameters"=w525:variant)
                n201 = Variant To Data(error in=w527, type=T29 {"Response Data"={"can_comm_state"={"fault_code"=0, "fault"=FALSE, "comm_state"=enum."Error_Active", "last_comm_error"=enum."None", "receive_error_counter"=0, "transmit_error_counter"=0, "transceiver_error"=FALSE, "sleep"=FALSE}, "frame"=[], "error"={"status"=FALSE, "code"=0, "source"=""}}, "Success"=FALSE} ("cluster"), Variant=w525) -> (data=w524:T29, error out=w528:errorcluster)
                n202 = Unbundle By Name(w524) -> ("Response Data.frame"=w523:T14[])
                n203 = call "LogEngine.LogFile.Write.vi"("error in (no error)"=w528, "Data"=w523, "Byte Stream File in"=w531) -> ("error out"=w530:errorcluster, "Byte Stream File out"=w529:refnum<file>)  [unwired: 7 in]
              }
            }
          }
        }
      }
      frame "Stop", "Exit" {
        # "Stop or Exit the subprocess."
        n204 = Not A Number/Path/Refnum?(number/path/refnum=w554) -> (NaN/Path/Refnum?=w555:bool)
        n205 = case shown="False" w555 {
          tunnel: w554 -> [w561 _]
          tunnel: w552 -> [w560 _]
          tunnel: [w557 _] -> w546
          frame False {
            # "Open log file. Close it and convert from .BIN to .TXT."
            n206 = property class="Str"(reference=w560, "Value"="Converting BIN file to TXT..") -> (reference out=w558:refnum<vi>, error out=w556:errorcluster)  [unwired: 1 in]
            n207 = flat-sequence {
              tunnel: w561 -> [w568]
              tunnel: w558 -> [w565]
              tunnel: [w564] -> w557
              tunnel: w556 -> [_]
              frame #0 {
                n208 = Close File(refnum=w568) -> (path=w563:path, error out=w562:errorcluster)  [unwired: 1 in]
                n209 = call "LogEngine.LogFile.Convert.vi"("error in (no error)"=w562, "path"=w563) -> ("error out"=w566:errorcluster, "Status"=w569:string)  [unwired: 8 in]
                n210 = property class="Str"(reference=w565, "Value"=w569) -> (error out=w567:errorcluster)  [unwired: 1 in, 1 out]
                n211 = Merge Errors(w567, w566) -> (w564:errorcluster)
              }
            }
          }
          frame True {
            # "No open log file. Do nothing."
          }
        }
        n212 = Equal?(x=SubProcessEngine.State."Exit", y=w547) -> (x = y?=w551:bool)
        n213 = Select(t=w547, s=w551, f=SubProcessEngine.State."Idle" ("x")) -> (s? t:f=w548:T6)
      }
    }
  }
  n214 = while {
    tunnel: w17 -> [w593]
    tunnel: w16 -> [w595]
    tunnel: [w594] -> w8
    shift-right: [w592] -> _
    shift-left: SubProcessEngine.State."Idle" ("State") -> [w587]
    tunnel: w9 -> [w591]
    shift-right: [w589] -> _
    shift-left: _ -> [w575]
    stop <- w588 stop-if-true
    # "Process Results Loop - Process the Bus Data/Status from the gRPC Stream loop based on User parameters and display results."
    n215 = call "SubProcessEngine.GetNextState.vi"("error in (no error)"=w591, "State"=w587, "timeout in ms (5)"=250, "Q"=w593) -> ("error out"=w577:errorcluster, "State"=w573:T6, "timed out?"=w586:bool, "Data"=w590:T30)  [unwired: 4 in]
    n216 = flat-sequence {
      tunnel: ["Pause"] -> w584
      tunnel: ["Type Filter"] -> w583
      tunnel: ["Direction Filter"] -> w582
      tunnel: ["Host Filter"] -> w581
      tunnel: ["Filter IDs"] -> w580
      tunnel: ["Clear History"] -> w579
      tunnel: ["Sort By ID"] -> w578
      tunnel: w577 -> [w599]
      tunnel: [w599] -> w576
      tunnel: w575 -> [w598]
      tunnel: [w598] -> w574
      tunnel: w573 -> [w597]
      tunnel: [w597] -> w572
      frame #0 {
      }
    }
    n217 = case shown="\"Process\"" w572 {
      selector: w572 -> [w613 _ _ _ w669]
      tunnel: w595 -> [w609 _ w644 w660 w664]
      tunnel: [w607 w614 w626 w655 w662] -> w594
      tunnel: [w613 SubProcessEngine.State."Process" ("State") SubProcessEngine.State."Process" ("State") SubProcessEngine.State."Idle" ("State") w669] -> w592
      tunnel: w576 -> [w608 w614 w640 w657 w663]
      tunnel: w590 -> [_ _ w642 _ _]
      tunnel: [_ TRUE _ _ _] -> w589
      tunnel: w574 -> [_ _ w630 _ _]
      tunnel: [_ _ _ _ TRUE] -> w588
      tunnel: w586 -> [_ _ w636 _ _]
      tunnel: w584 -> [_ _ w625 _ _]
      tunnel: w583 -> [_ _ w624 _ _]
      tunnel: w582 -> [_ _ w623 _ _]
      tunnel: w581 -> [_ _ w622 _ _]
      tunnel: w580 -> [_ _ w621 _ _]
      tunnel: w579 -> [_ _ w620 _ _]
      tunnel: w578 -> [_ _ w619 _ _]
      tunnel: [_ _ w618 _ _] -> w571
      tunnel: [_ _ w617 _ _] -> w570
      frame "Idle" {
        # "Do Nothing."
        n218 = property class="Str"(reference=w609, "Value"="Bus: Idle..", "Blinking"=FALSE) -> (error out=w610:errorcluster)  [unwired: 1 in, 1 out]
        n219 = Merge Errors(w610, w608) -> (w607:errorcluster)
      }
      frame "Arm" {
        # "Set the re-init flag and go to the next state."
      }
      frame "Process" {
        # "Handle bus data. Allowing timeouts is required so user parameters are applied, even if new data is not available."
        n220 = Unbundle By Name(w642) -> ("Parameters"=w641:variant)
        n221 = call "Convert.StringToArray.vi"("Filter IDs"=w621) -> ("Filter IDs"=w634:u32[])  [unwired: 10 in]
        n222 = Variant To Data(error in=w640, type=T29 {"Response Data"={"can_comm_state"={"fault_code"=0, "fault"=FALSE, "comm_state"=enum."Error_Active", "last_comm_error"=enum."None", "receive_error_counter"=0, "transmit_error_counter"=0, "transceiver_error"=FALSE, "sleep"=FALSE}, "frame"=[], "error"={"status"=FALSE, "code"=0, "source"=""}}, "Success"=FALSE} ("cluster"), Variant=w641) -> (data=w639:T29, error out=w629:errorcluster)
        n223 = Bundle By Name(cluster=T32 {"Host Filter"=FALSE, "Filter Parameters"={"filter_ids"=[], "direction_filter"=enum."TX_RX", "frame_filter"=enum."CAN_Data"}, "Sort By ID"=FALSE, "Pause"=FALSE, "Clear History"=FALSE} ("Host Parameters"), "Clear History"=w620, "Pause"=w625, "Sort By ID"=w619, "Filter Parameters.direction_filter"=w623, "Filter Parameters.frame_filter"=w624, "Host Filter"=w622, "Filter Parameters.filter_ids"=w634) -> (w631:T32)
        n224 = Unbundle By Name(w639) -> ("Response Data.can_comm_state"=w637:T26, "Success"=w632:bool, "Response Data.frame"=w638:T14[])
        n225 = case shown="False" w636 {
          tunnel: w644 -> [w653 _]
          tunnel: [w649 w654] -> w628
          tunnel: w637 -> [w648 _]
          tunnel: w632 -> [w646 _]
          tunnel: w629 -> [w645 w654]
          frame False {
            # "Process Comm State"
            n226 = call "StreamEngine.Main.Stream.BusStatus.Process.vi"("error in (no error)"=w645, "Stream Connection"=w646, "State"=w648) -> ("error out"=w650:errorcluster, "Warning"=w652:bool, "State"=w647:string)  [unwired: 6 in]
            n227 = property class="Str"(reference=w653, "Value"=w647, "Blinking"=w652) -> (error out=w651:errorcluster)  [unwired: 1 in, 1 out]
            n228 = Merge Errors(w651, w650) -> (w649:errorcluster)
          }
          frame True {
            # "Timeout. Do nothing."
          }
        }
        n229 = call "StreamEngine.Main.Stream.BusData.Process.vi"("error in (no error)"=w629, "Host Parameters"=w631, "Init?"=w630, "frame"=w638) -> ("error out"=w627:errorcluster, "Table Update"=w618:bool, "Table"=w617:string[][])  [unwired: 5 in]
        n230 = Merge Errors(w628, w627) -> (w626:errorcluster)
      }
      frame "Stop" {
        # "Stop the data processing loop."
        n231 = property class="Str"(reference=w660, "Value"="Bus: Stopping..", "Blinking"=FALSE) -> (error out=w656:errorcluster)  [unwired: 1 in, 1 out]
        n232 = Merge Errors(w656, w657) -> (w655:errorcluster)
      }
      frame "Exit" {
        # "Exit the data processing loop."
        n233 = property class="Str"(reference=w664, "Value"="Bus: Exiting..", "Blinking"=FALSE) -> (error out=w665:errorcluster)  [unwired: 1 in, 1 out]
        n234 = Merge Errors(w665, w663) -> (w662:errorcluster)
      }
    }
    n235 = case shown="True" w571 {
      tunnel: w570 -> [_ w596]
      frame False {
      }
      frame True {
        "Table Control" <- w596
      }
    }
  }
  n236 = while {
    shift-right: [w679] -> _
    shift-left: StreamEngine.State."Wait" -> [w671]
    tunnel: w9 -> [w680]
    shift-right: [w678] -> _
    shift-left: T5 0 ("Call ID") -> [w677]
    tunnel: w19 -> [w675]
    tunnel: [w674] -> w18
    tunnel: w14 -> [w672]
    stop <- w676 stop-if-true
    # "gRPC Stream Loop - Begin, Read, and End the gRPC Stream for Bus Data/Status"
    n237 = call "StreamEngine.GetNextStreamState.vi"("error in (no error)"=w680, "Bus State"=w671, "Cmd Q"=w675) -> ("error out"=w681:errorcluster, "Bus State"=w670:T7, "Command Cluster"=w682:T33)  [unwired: 5 in, 1 out]
    n238 = case shown="\"Start Stream\"" w670 {
      selector: w670 -> [w683 _ w701 _ w712]
      tunnel: w681 -> [w684 w687 w698 w707 w714]
      tunnel: w682 -> [_ w690 _ _ _]
      tunnel: [w684 w688 w696 w705 w711] -> w674
      tunnel: [_ w689 w697 _ _] -> w678
      tunnel: w677 -> [_ _ w699 w706 w713]
      tunnel: [w683 w691 w700 StreamEngine.State."Wait" w712] -> w679
      tunnel: [_ _ _ w704 w710] -> w676
      tunnel: [_ _ w695 _ _] -> w673
      tunnel: w672 -> [_ w686 w694 w703 w709]
      frame "Wait", Default {
        # "Do Nothing"
      }
      frame "Start Stream" {
        # "Begin gRPC Stream"
        n239 = Unbundle By Name(w690) -> ("Parameters"=w685:variant)
        n240 = call "StreamEngine.Main.Stream.Start.vi"("Stream.Qs.SubProcesses"=w686, "error in (no error)"=w687, "Parameters"=w685) -> ("error out"=w688:errorcluster, "Stream Ref"=w689:T5)  [unwired: 6 in, 1 out]
        n241 = Select(t=StreamEngine.State."Stop Stream", s=w688, f=StreamEngine.State."Read Stream") -> (s? t:f=w691:T7)
      }
      frame "Read Stream" {
        # "Read Data from gRPC Stream"
        n242 = call "StreamEngine.Main.Stream.Read.vi"("error in (no error)"=w698, "SubProcesses"=w694, "gRPC ID"=w699) -> ("error out"=w696:errorcluster, "Success"=w695:bool, "gRPC ID out"=w697:T5)  [unwired: 6 in]
        n243 = Select(t=StreamEngine.State."Stop Stream", s=w696, f=w701) -> (s? t:f=w700:T7)
      }
      frame "Stop Stream" {
        w704 = FALSE ("Exit?")
        # "Close gRPC Stream"
        n244 = call "StreamEngine.Main.Stream.Stop.vi"("error in (no error)"=w707, "Exit?"=w704, "Stream.Qs.SubProcesses"=w703, "Stream Ref"=w706) -> ("error out"=w705:errorcluster)  [unwired: 7 in]
      }
      frame "Exit" {
        w710 = TRUE
        # "Exit Loop"
        n245 = call "StreamEngine.Main.Stream.Stop.vi"("error in (no error)"=w714, "Exit?"=w710, "Stream.Qs.SubProcesses"=w709, "Stream Ref"=w713) -> ("error out"=w711:errorcluster)  [unwired: 7 in]
      }
    }
    "Stream Connected" <- w673
  }
  n246 = flat-sequence {
    tunnel: w42 -> [w720]
    tunnel: w18 -> [w718]
    tunnel: w8 -> [w717]
    tunnel: w7 -> [w719]
    tunnel: w6 -> [w716]
    tunnel: [w715] -> w1
    frame #0 {
      n247 = call "GUI.Close.vi"("State Variables in"=w720) -> ()  [unwired: 11 in]
      n248 = Merge Errors(w719, w718, w717, w716) -> (w715:errorcluster)
    }
  }
  "error out" <- w1
